vi "Update Time table.vi"(8 "error in (no error)":errorcluster, 10 "Time table (Second)":T1, 11 "Configuration Database Actor in":refnum<class "Configuration Database Actor.lvclass">) -> (0 "error out":errorcluster, 3 "Configuration Database Actor out":refnum<class "Configuration Database Actor.lvclass">)   [LabVIEW 2022 SP3, in "Configuration Database Actor.lvlib" / "Configuration Database Actor.lvclass"]
uses:
  Configuration Database Actor.lvclass
  Time Table.ctl
  Configuration Database Actor.lvclass/Configuration Database Actor.ctl
panel:
  # "[Covers: CD4]"
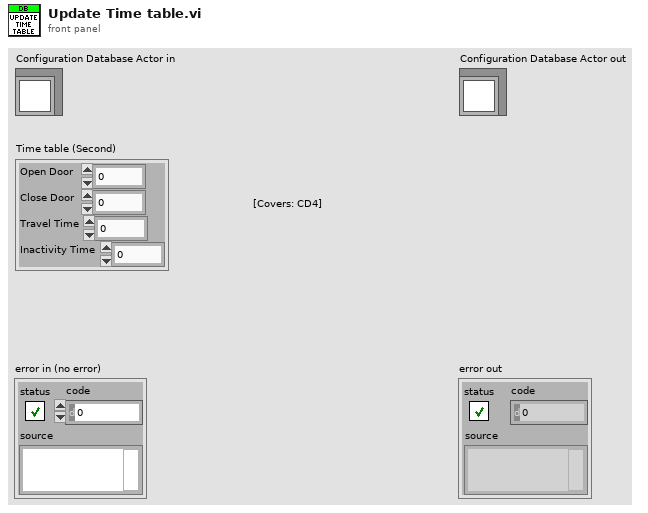
[diagram p1: front panel]
types:
  T1 = typedef "Configuration Database Actor.lvlib/Configuration Database Actor.lvclass/Time Table.ctl" = cluster{"Open Door":u32, "Close Door":u32, "Travel Time":u32, "Inactivity Time":u32}
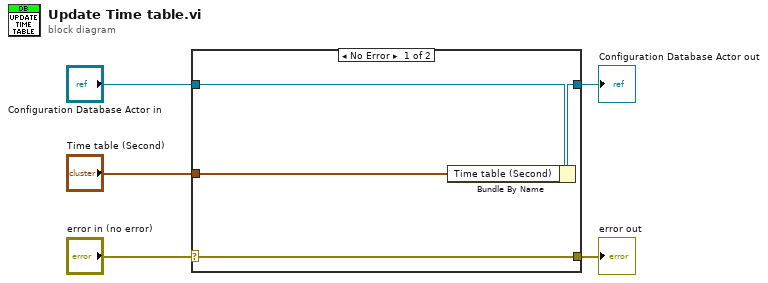
[diagram p0: block diagram]
diagram:
  n1 = case shown="No Error" "error in (no error)" {
    selector: "error in (no error)" -> [w9 w10]
    tunnel: [w9 w10] -> w4
    tunnel: [w7 w11] -> w2
    tunnel: "Configuration Database Actor in" -> [w8 w11]
    tunnel: "Time table (Second)" -> [w6 _]
    frame No Error {
      n2 = Bundle By Name(cluster=w8, "Time table (Second)"=w6) -> (w7:refnum<class "Configuration Database Actor.lvclass">)
    }
    frame Error {
    }
  }
  "error out" <- w4
  "Configuration Database Actor out" <- w2
